vi "管理用户.vi"() -> ()   [LabVIEW 2018]
uses:
  <vilib>/Utility/file.llb/Read Delimited Spreadsheet (string).vi
  <vilib>/Utility/file.llb/Write Delimited Spreadsheet (string).vi
panel:
  in  "所选密码":string
  in  "所选用户名":string
  in  "修改用户":bool
  out "新值":i32
  in  "删除用户":bool
  in  "添加用户":bool
  in  "多列列表框":i32(listbox)
  in  "退出管理":bool
  # "管理用户系统"
  # "注：修改或删除用户信息请先选中所在行"
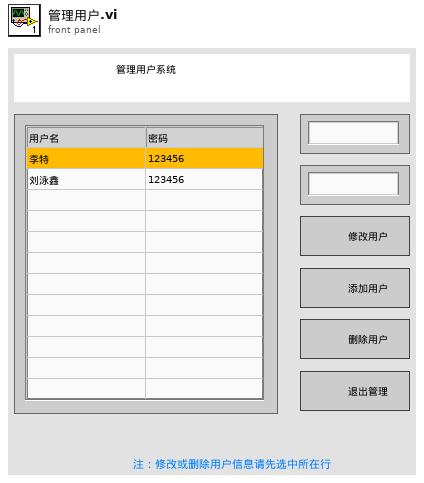
[diagram p1: front panel]
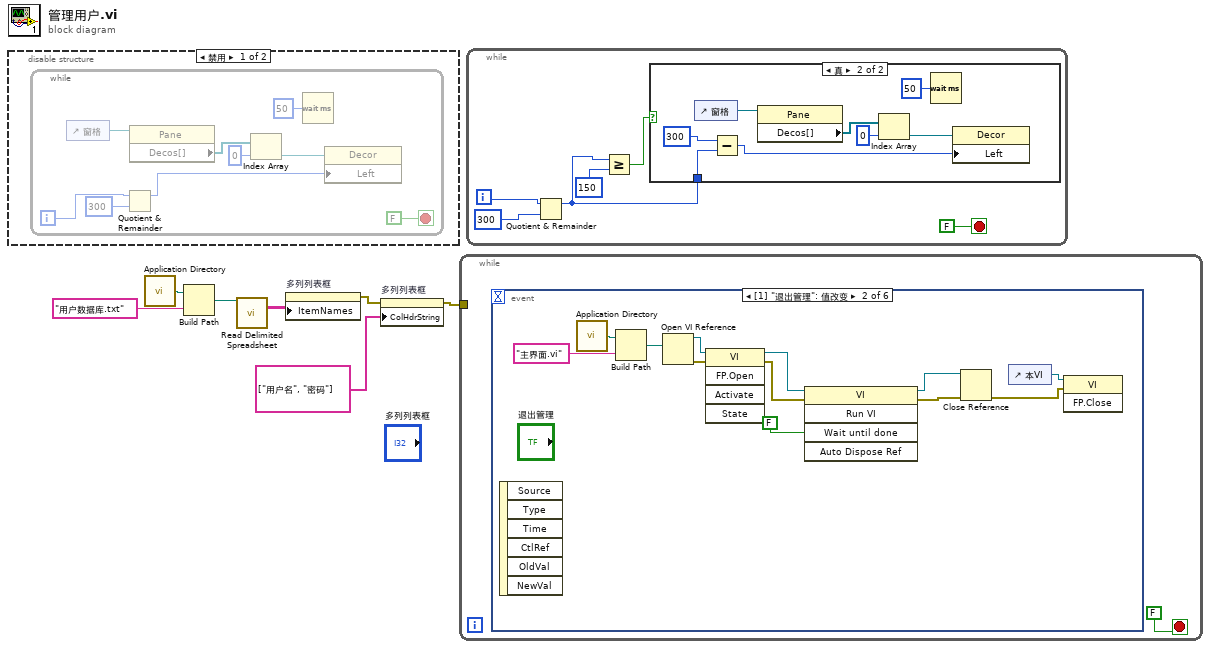
[diagram p0: block diagram]
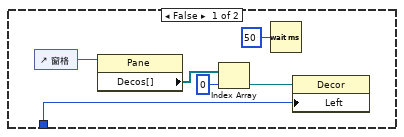
[diagram p3: hidden frame]
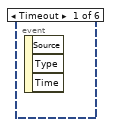
[diagram p4: hidden frame]
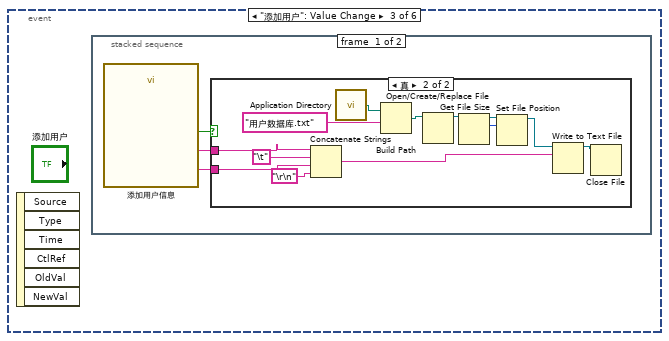
[diagram p5: hidden frame]
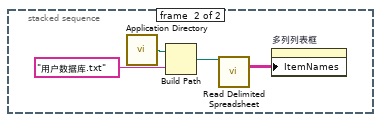
[diagram p7: hidden frame]
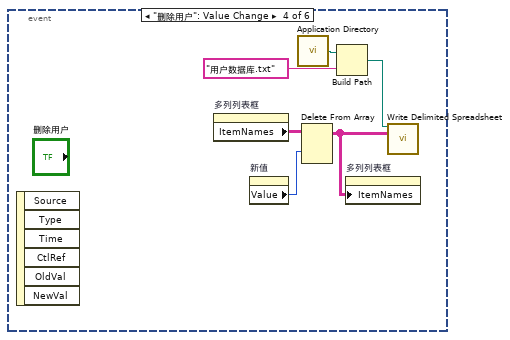
[diagram p8: hidden frame]
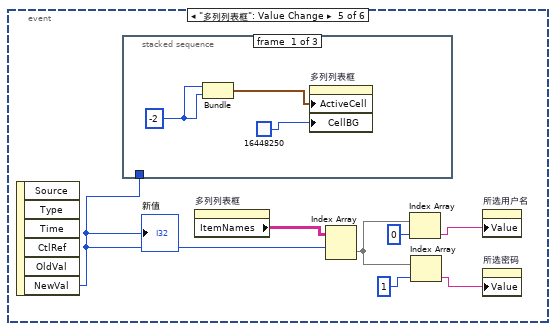
[diagram p9: hidden frame]
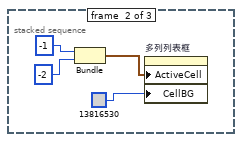
[diagram p10: hidden frame]
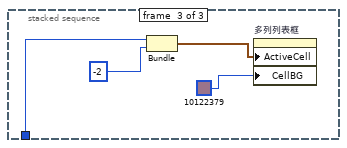
[diagram p11: hidden frame]
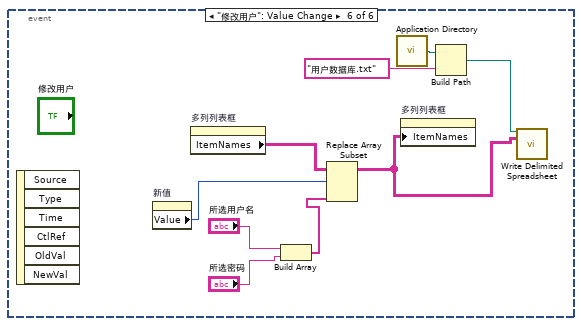
[diagram p12: hidden frame]
diagram:
  n1 = disable-structure shown="禁用" {
    frame Disabled {
      n2 = while {
        i -> [w11]
        stop <- FALSE stop-if-true
        n3 = control-ref of="窗格"() -> (w16:refnum<vi>)
        n4 = Quotient & Remainder(x=w11, y=300) -> (x-y*floor(x/y)=w9:i32)  [unwired: 1 out]
        n5 = property class="Pane"(reference=w16) -> ("Decos[]"=w15:refnum<vi>[])  [unwired: 1 in, 2 out]
        n6 = Index Array(array=w15, index=0 ("索引")) -> (element=w13:refnum<vi>)
        n7 = Wait (ms)(milliseconds to wait=u32 50 ("等待时间（毫秒）")) -> ()  [unwired: 1 out]
        n8 = property class="Decor"(reference=w13, "Left"=w9) -> ()  [unwired: 1 in, 2 out]
      }
    }
    frame Enabled {
    }
  }
  n9 = call <vilib>:"Application Directory.vi"() -> ("Application Directory"=w7:path)
  n10 = Build Path(base path=w7, name or relative path="用户数据库.txt" ("名称或相对路径")) -> (appended path=w6:path)
  n11 = call-poly <vilib>:"Read Delimited Spreadsheet.vi"("file path (dialog if empty)"=w6) -> ("all rows"=w4:string[][])  [unwired: 9 in, 5 out]
  n12 = property on="多列列表框" class="MCListbox (严格)"("ItemNames"=w4) -> (error out=w2:errorcluster)  [unwired: 2 in, 1 out]
  n13 = property on="多列列表框" class="MCListbox (严格)"(error in=w2, "ColHdrString"=string[] ["用户名", "密码"] ("列首字符串[]")) -> (error out=w1:errorcluster)  [unwired: 1 in, 1 out]
  n14 = while {
    tunnel: w1 -> [_]
    stop <- FALSE stop-if-true
    n15 = event shown="[1] \"退出管理\": 值改变" {
      selector: _ -> [_ _ _ _ _ _]
      dyn-events: _ -> [_ _ _ _ _ _]
      timeout: _ -> [_ _ _ _ _ _]
      event Timeout {
        n16 = event-data() -> ()  [unwired: 1 in, 3 out]
      }
      event "退出管理": Value Change {
        n17 = event-data() -> ()  [unwired: 1 in, 6 out]
        n18 = call <vilib>:"Application Directory.vi"() -> ("Application Directory"=w28:path)
        n19 = Build Path(base path=w28, name or relative path="主界面.vi" ("名称或相对路径")) -> (appended path=w29:path)
        n20 = Open VI Reference(vi path=w29) -> (vi reference=w26:refnum<vi>, error out=w25:errorcluster)  [unwired: 5 in]
        n21 = invoke class="VI" method="FP.Open"(reference=w26, error in=w25) -> (reference out=w24:refnum<vi>, error out=w23:errorcluster)  [unwired: 3 in, 3 out]
        n22 = invoke class="VI" method="Run VI"(reference=w24, error in=w23, "Wait until done"=FALSE ("结束前等待")) -> (reference out=w20:refnum<vi>, error out=w21:errorcluster)  [unwired: 2 in, 3 out]
        n23 = Close Reference(reference=w20, error in (no error)=w21) -> (error out=w18:errorcluster)
        n24 = control-ref of="本VI"() -> (w19:refnum<vi>)
        n25 = invoke class="VI" method="FP.Close"(reference=w19, error in=w18) -> ()  [unwired: 1 in, 3 out]
      }
      event "添加用户": Value Change {
        n26 = event-data() -> ()  [unwired: 1 in, 6 out]
        n27 = stacked-sequence {
          frame #0 {
            n28 = call "添加用户信息"() -> ("密码"=w31:string, "用户名"=w32:string, "添加用户"=w30:bool)  [unwired: 16 in, 1 out]
            n29 = case shown="真" w30 {
              tunnel: w32 -> [_ w38]
              tunnel: w31 -> [_ w36]
              frame False {
              }
              frame True {
                n30 = Concatenate Strings(w38, "\t", w36, "\r\n") -> (w34:string)
                n31 = call <vilib>:"Application Directory.vi"() -> ("Application Directory"=w44:path)
                n32 = Build Path(base path=w44, name or relative path="用户数据库.txt" ("名称或相对路径")) -> (appended path=w43:path)
                n33 = Open/Create/Replace File(file path (use dialog)=w43) -> (refnum out=w42:refnum<file>)  [unwired: 5 in, 2 out]
                n34 = Get File Size(file=w42) -> (refnum out=w33:refnum<file>, size (in bytes)=w41:i64)  [unwired: 1 in, 1 out]
                n35 = Set File Position(offset (in bytes) (0)=w41, refnum=w33) -> (refnum out=w40:refnum<file>)  [unwired: 2 in, 1 out]
                n36 = Write to Text File(file (use dialog)=w40, text=w34) -> (refnum out=w39:refnum<file>)  [unwired: 2 in, 2 out]
                n37 = Close File(refnum=w39) -> ()  [unwired: 1 in, 2 out]
              }
            }
          }
          frame #1 {
            n38 = call <vilib>:"Application Directory.vi"() -> ("Application Directory"=w49:path)
            n39 = Build Path(base path=w49, name or relative path="用户数据库.txt" ("名称或相对路径")) -> (appended path=w48:path)
            n40 = call-poly <vilib>:"Read Delimited Spreadsheet.vi"("file path (dialog if empty)"=w48) -> ("all rows"=w47:string[][])  [unwired: 9 in, 5 out]
            n41 = property on="多列列表框" class="MCListbox (严格)"("ItemNames"=w47) -> ()  [unwired: 2 in, 2 out]
          }
        }
      }
      event "删除用户": Value Change {
        n42 = event-data() -> ()  [unwired: 1 in, 6 out]
        n43 = property on="多列列表框" class="MCListbox (严格)"() -> ("ItemNames"=w55:string[][])  [unwired: 2 in, 2 out]
        n44 = property on="新值" class="DigNum (严格)"() -> ("Value"=w54:i32)  [unwired: 2 in, 2 out]
        n45 = call <vilib>:"Application Directory.vi"() -> ("Application Directory"=w52:path)
        n46 = Delete From Array(array=w55, index (row)=w54) -> (array with subset deleted=w50:string[][])  [unwired: 2 in, 1 out]
        n47 = Build Path(base path=w52, name or relative path="用户数据库.txt" ("名称或相对路径")) -> (appended path=w51:path)
        n48 = property on="多列列表框" class="MCListbox (严格)"("ItemNames"=w50) -> ()  [unwired: 2 in, 2 out]
        n49 = call-poly <vilib>:"Write Delimited Spreadsheet.vi"("file path (dialog if empty)"=w51, "2D data"=w50) -> ()  [unwired: 12 in, 2 out]
      }
      event "多列列表框": Value Change {
        n50 = event-data() -> ("NewVal"=w61:i32)  [unwired: 1 in, 5 out]
        "新值" <- w61
        n51 = stacked-sequence {
          tunnel: w61 -> [_ _ w73]
          frame #0 {
            w63 = -2
            n52 = Bundle(w63, w63) -> (w64:cluster{i32, i32})  [unwired: 1 in]
            n53 = property on="多列列表框" class="MCListbox (严格)"("ActiveCell"=w64, "CellBG"=u32 16448250) -> ()  [unwired: 2 in, 2 out]
          }
          frame #1 {
            n54 = Bundle(-1, -2) -> (w66:cluster{i32, i32})  [unwired: 1 in]
            n55 = property on="多列列表框" class="MCListbox (严格)"("ActiveCell"=w66, "CellBG"=u32 13816530) -> ()  [unwired: 2 in, 2 out]
          }
          frame #2 {
            n56 = Bundle("NewVal"=w73, -2) -> (w71:cluster{"NewVal":i32, i32})  [unwired: 1 in]
            n57 = property on="多列列表框" class="MCListbox (严格)"("ActiveCell"=w71, "CellBG"=u32 10122379) -> ()  [unwired: 2 in, 2 out]
          }
        }
        n58 = property on="多列列表框" class="MCListbox (严格)"() -> ("ItemNames"=w62:string[][])  [unwired: 2 in, 2 out]
        n59 = Index Array(array=w62, index (row)=w61) -> (element=w60:string[])  [unwired: 1 in]
        n60 = Index Array(array=w60, index=0 ("索引")) -> (element=w57:string)
        n61 = Index Array(array=w60, index=1 ("索引")) -> (element=w56:string)
        n62 = property on="所选用户名" class="Str"("Value"=w57) -> ()  [unwired: 2 in, 2 out]
        n63 = property on="所选密码" class="Str"("Value"=w56) -> ()  [unwired: 2 in, 2 out]
      }
      event "修改用户": Value Change {
        n64 = event-data() -> ()  [unwired: 1 in, 6 out]
        n65 = property on="新值" class="DigNum (严格)"() -> ("Value"=w81:i32)  [unwired: 2 in, 2 out]
        n66 = property on="多列列表框" class="MCListbox (严格)"() -> ("ItemNames"=w82:string[][])  [unwired: 2 in, 2 out]
        n67 = Build Array("所选用户名", "所选密码") -> (w74:string[])
        n68 = Replace Array Subset(array=w82, new element=w74, index (row)=w81) -> (w78:string[][])  [unwired: 1 in]
        n69 = call <vilib>:"Application Directory.vi"() -> ("Application Directory"=w80:path)
        n70 = property on="多列列表框" class="MCListbox (严格)"("ItemNames"=w78) -> ()  [unwired: 2 in, 2 out]
        n71 = Build Path(base path=w80, name or relative path="用户数据库.txt" ("名称或相对路径")) -> (appended path=w79:path)
        n72 = call-poly <vilib>:"Write Delimited Spreadsheet.vi"("file path (dialog if empty)"=w79, "2D data"=w78) -> ()  [unwired: 12 in, 2 out]
      }
    }
  }
  n73 = while {
    i -> [w87]
    stop <- FALSE stop-if-true
    n74 = Quotient & Remainder(x=w87, y=300) -> (x-y*floor(x/y)=w83:i32)  [unwired: 1 out]
    n75 = Greater Or Equal?(x=w83, y=150) -> (x >= y?=w84:bool)
    n76 = case shown="真" w84 {
      tunnel: w83 -> [w89 w96]
      frame False {
        n77 = control-ref of="窗格"() -> (w94:refnum<vi>)
        n78 = property class="Pane"(reference=w94) -> ("Decos[]"=w93:refnum<vi>[])  [unwired: 1 in, 2 out]
        n79 = Index Array(array=w93, index=0 ("索引")) -> (element=w92:refnum<vi>)
        n80 = Wait (ms)(milliseconds to wait=u32 50 ("等待时间（毫秒）")) -> ()  [unwired: 1 out]
        n81 = property class="Decor"(reference=w92, "Left"=w89) -> ()  [unwired: 1 in, 2 out]
      }
      frame True {
        n82 = control-ref of="窗格"() -> (w102:refnum<vi>)
        n83 = Subtract(x=300 ("y"), y=w96) -> (x-y=w95:i32)
        n84 = property class="Pane"(reference=w102) -> ("Decos[]"=w101:refnum<vi>[])  [unwired: 1 in, 2 out]
        n85 = Index Array(array=w101, index=0 ("索引")) -> (element=w99:refnum<vi>)
        n86 = Wait (ms)(milliseconds to wait=u32 50 ("等待时间（毫秒）")) -> ()  [unwired: 1 out]
        n87 = property class="Decor"(reference=w99, "Left"=w95) -> ()  [unwired: 1 in, 2 out]
      }
    }
  }
